vi "ControlIndexForChannel.vi"(7 "Full Path":bool, 8 "error in (no error)":errorcluster, 9 "Versitand Channels":T1[](array[typedef]), 10 "Control Names":string[](array[string]), 11 "Controls References":refnum<vi>[](array[refnum])) -> (0 "error out":errorcluster, 1 "Channel Name":string[](array[string]), 2 "Control Index":i32[](array[numeric]))   [LabVIEW 2017]
uses:
  <vilib>/NI Veristand/Execution/Workspace/NodeInfo.ctl
  <vilib>/NI Veristand/Execution/Workspace/Waveform Data Type.ctl
  <vilib>/NI Veristand/Execution/Workspace/NI_VS Workspace ExecutionAPI.lvlib
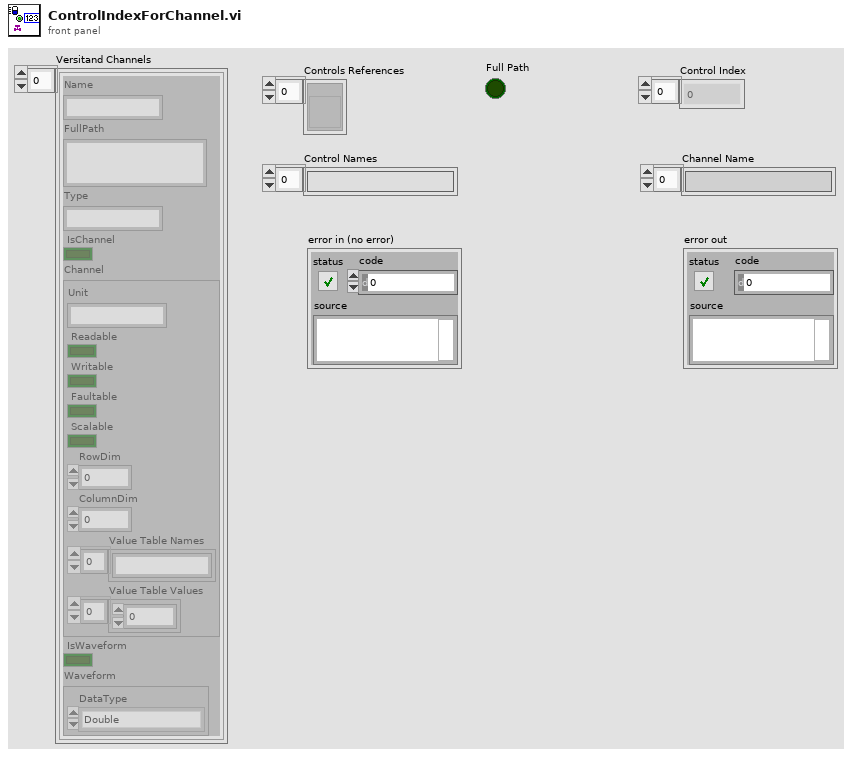
[diagram p1: front panel]
types:
  T1 = typedef "NI_VS Workspace ExecutionAPI.lvlib/NodeInfo.ctl" = cluster{"Name":string, "FullPath":string, "Type":string, "IsChannel":bool, "Channel":cluster{"Unit":string, "Readable":bool, "Writable":bool, "Faultable":bool, "Scalable":bool, "RowDim":u32, "ColumnDim":u32, "Value Table Names":string[], "Value Table Values":dbl[]}, "IsWaveform":bool, "Waveform":cluster{"DataType":T2}}
  T2 = typedef "NI_VS Workspace ExecutionAPI.lvlib/Waveform Data Type.ctl" = enum16{"Double", "ComplexDouble"}
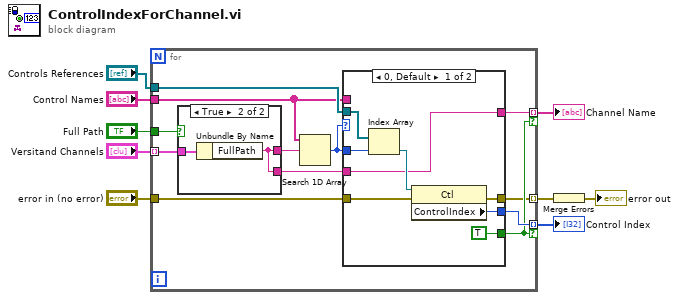
[diagram p0: block diagram]
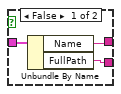
[diagram p2: hidden frame]
diagram:
  n1 = for {
    tunnel: "Versitand Channels" -> [w21] mode=indexing
    tunnel: "Control Names" -> [w18]
    tunnel: "Controls References" -> [w19]
    tunnel: [w16] -> w5 mode=indexing if=w14
    tunnel: [w17] -> w4 mode=indexing if=w14
    tunnel: "error in (no error)" -> [w13]
    tunnel: [w12] -> w8 mode=indexing
    tunnel: "Full Path" -> [w11]
    n2 = case shown="True" w11 {
      tunnel: w21 -> [w24 w26]
      tunnel: [w23 w25] -> w20
      tunnel: [w22 w25] -> w10
      frame False {
        n3 = Unbundle By Name(w24) -> ("Name"=w23:string, "FullPath"=w22:string)
      }
      frame True {
        n4 = Unbundle By Name(w26) -> ("FullPath"=w25:string)
      }
    }
    n5 = Search 1D Array(1D array=w18, element=w20) -> (index of element=w15:i32)  [unwired: 1 in]
    n6 = case shown="0, Default" w15 {
      tunnel: w19 -> [w34 _]
      tunnel: w18 -> [_ _]
      tunnel: w15 -> [w33 _]
      tunnel: [w27 _] -> w17
      tunnel: [w31 _] -> w16
      tunnel: [TRUE _] -> w14
      tunnel: w13 -> [w29 w35]
      tunnel: [w28 w35] -> w12
      tunnel: w10 -> [w27 _]
      frame 0, Default {
        n7 = Index Array(array=w34, index=w33) -> (element=w32:refnum<vi>)
        n8 = property class="Ctl"(reference=w32, error in=w29) -> (error out=w28:errorcluster, "ControlIndex"=w31:i32)  [unwired: 1 out]
      }
      frame -1 {
      }
    }
  }
  "Control Index" <- w5
  "Channel Name" <- w4
  n9 = Merge Errors(w8) -> (→"error out":errorcluster)
